vi "Unpack Variant Value.vi"(11 "VariantValueMsg in":refnum<class "VariantValueMsg.lvclass">) -> (2 "Value":variant, 3 "Name":string)   [LabVIEW 2015, in "ActorAutoRegistration.lvlib" / "VariantValueMsg.lvclass"]
uses:
  VariantValueMsg.lvclass
  VariantValueMsg.lvclass/VariantValueMsg.ctl
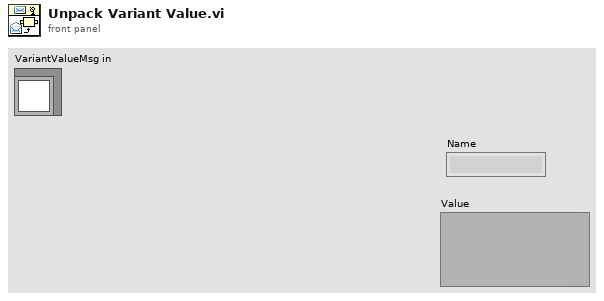
[diagram p1: front panel]
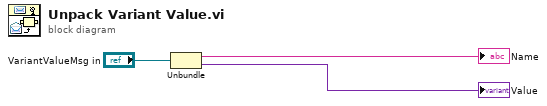
[diagram p0: block diagram]
diagram:
  n1 = Unbundle("VariantValueMsg in") -> (→"Name":string, →"Value":variant)
